vi "Activity 2-2 Program Architecture for Simple AAV.vi"() -> ()   [LabVIEW 2015]
panel:
  in  "Frequency":dbl(knob)=400.0 min=400.0 max=1600.0 step=100.0 scale=400.0..1600.0
  out "Average Value":dbl
  out "Waveform Graph":dynamicdata(graph)
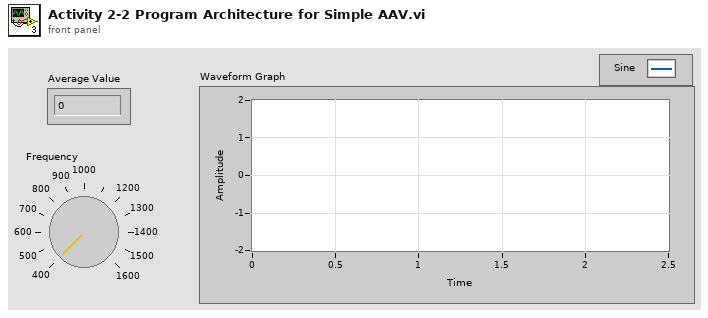
[diagram p1: front panel]
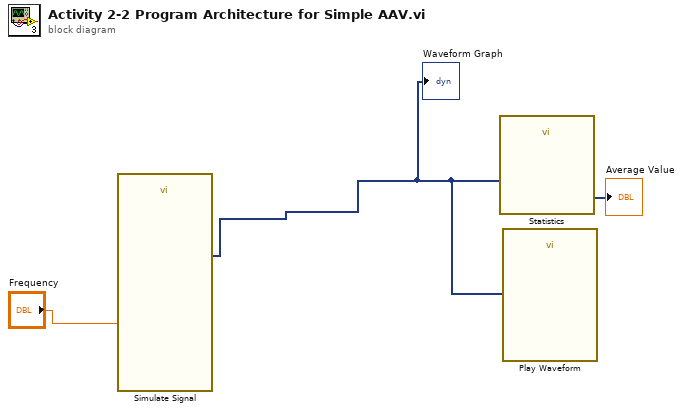
[diagram p0: block diagram]
diagram:
  n1 = call "Simulate Signal"("Frequency"="Frequency") -> ("Sine"=w1:dynamicdata)  [unwired: 13 in, 1 out]
  "Waveform Graph" <- w1
  n2 = call "Statistics"("Signals"=w1) -> ("Arithmetic Mean"=→"Average Value":dynamicdata)  [unwired: 25 in, 1 out]
  n3 = call "Play Waveform"("Data"=w1) -> ()  [unwired: 18 in, 1 out]
